vi "Print Report_ABB.vi"(11 "Report  path":path) -> ()   [LabVIEW 2017]
uses:
  ABB global.vi
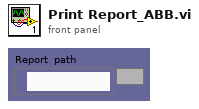
[diagram p1: front panel]
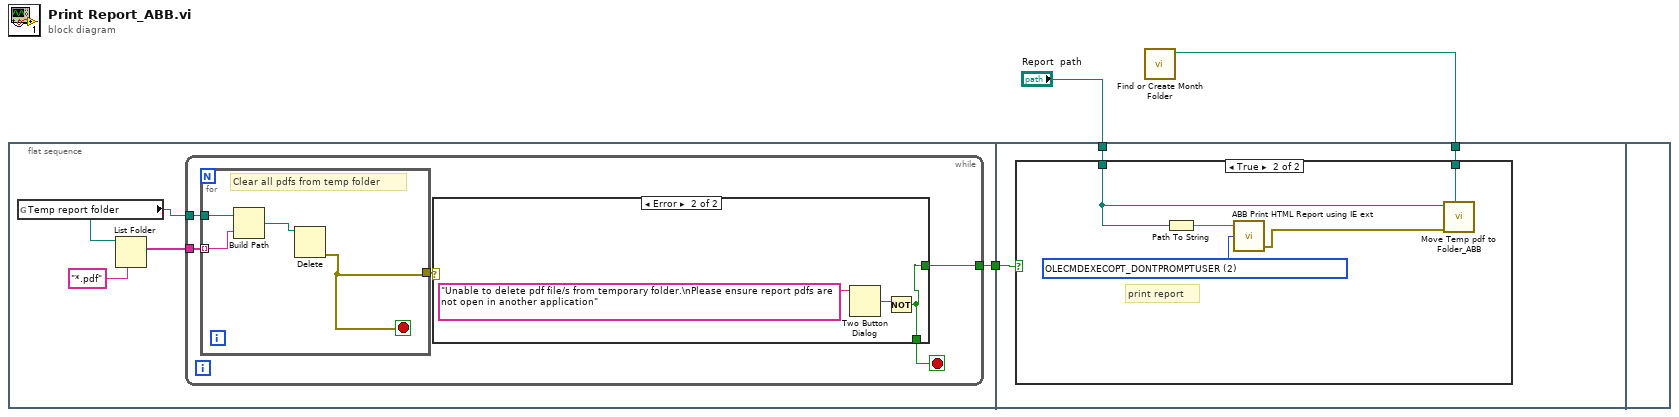
[diagram p0: block diagram]
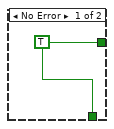
[diagram p2: hidden frame]
diagram:
  n1 = flat-sequence {
    tunnel: [w4] -> w2
    tunnel: "Report  path" -> [w23]
    tunnel: w2 -> [w22]
    tunnel: w1 -> [w21]
    frame #0 {
      n2 = global read "ABB global.vi" "Temp report folder"() -> (w5:path)
      n3 = List Folder(path=w5, pattern="*.pdf") -> (filenames=w6:string[])  [unwired: 2 in, 3 out]
      n4 = while {
        tunnel: w6 -> [w12]
        tunnel: w5 -> [w11]
        tunnel: [w8] -> w4
        stop <- w9 stop-if-true
        n5 = for {
          tunnel: w12 -> [w19] mode=indexing
          tunnel: w11 -> [w20]
          tunnel: [w17] -> w10
          stop <- w17 stop-if-true
          # "Clear all pdfs from temp folder"
          n6 = Build Path(base path=w20, name or relative path=w19) -> (appended path=w18:path)
          n7 = Delete(path (use dialog)=w18) -> (error out=w17:errorcluster)  [unwired: 4 in, 2 out]
        }
        n8 = case shown="Error" w10 {
          tunnel: [w13 w14] -> w9
          tunnel: [w13 w14] -> w8
          frame No Error {
            w13 = TRUE
          }
          frame Error {
            n9 = Two Button Dialog(message="Unable to delete pdf file/s from temporary folder.\nPlease ensure report pdfs are not open in another application") -> (T button?=w15:bool)  [unwired: 2 in]
            n10 = Not(x=w15) -> (.not. x?=w14:bool)
          }
        }
      }
    }
    frame #1 {
      n11 = case shown="True" w22 {
        tunnel: w23 -> [_ w25]
        tunnel: w21 -> [_ w24]
        frame False {
        }
        frame True {
          w28 = 2 items=["OLECMDEXECOPT_DODEFAULT", "OLECMDEXECOPT_PROMPTUSER", "OLECMDEXECOPT_DONTPROMPTUSER", "OLECMDEXECOPT_SHOWHELP"] ("IE Print Options")
          # "print report"
          n12 = Path To String(path=w25) -> (string=w27:string)
          n13 = call "ABB Print HTML Report using IE ext.vi"("IE Print Options"=w28, "Path to HTML"=w27) -> ("Error Out"=w26:errorcluster)  [unwired: 3 in]
          n14 = call "Move Temp pdf to Folder_ABB.vi"("Month Folder"=w24, "error in (no error)"=w26, "Report  path"=w25) -> ()  [unwired: 9 in]
        }
      }
    }
    frame #2 {
    }
  }
  n15 = call "Find or Create Month Folder.vi"() -> ("Month Folder"=w1:path)  [unwired: 11 in]
